vi "PXI-Can Resume From Error.vi"(0 "Ignore local?":bool, 7 "Abort":bool, 11 "error in (no error)":errorcluster) -> (4 "code":i32, 8 "Resume?":bool, 15 "error out":errorcluster)   [LabVIEW 2020]
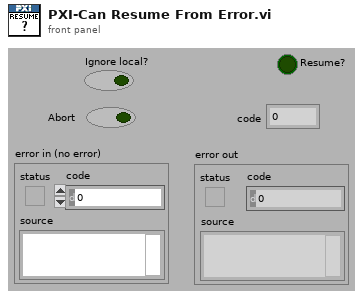
[diagram p1: front panel]
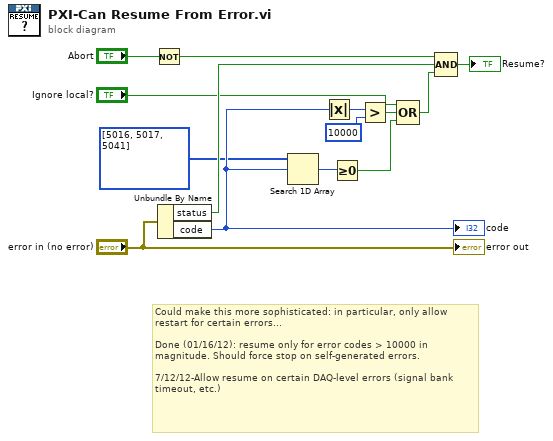
[diagram p0: block diagram]
diagram:
  # "Could make this more sophisticated: in particular, only allow restart for certain errors...\n\nDone (01/16/12): resume only for error codes > 10000 in magnitude. Should force stop on self-generated errors.\n\n7/12/12-Allow resume on certain DAQ-level errors (signal bank timeout, etc.)"
  n1 = Not(x="Abort") -> (.not. x?=w11:bool)
  n2 = Unbundle By Name("error in (no error)") -> ("status"=w12:bool, "code"=w4:i32)
  "code" <- w4
  n3 = Search 1D Array(1D array=i32[] [5016, 5017, 5041], element=w4) -> (index of element=w3:i32)  [unwired: 1 in]
  n4 = Absolute Value(x=w4) -> (abs(x)=w9:i32)
  n5 = Greater Or Equal To 0?(x=w3) -> (x >= 0?=w2:bool)
  n6 = Greater?(x=w9, y=10000) -> (0:w7:bool)
  n7 = Compound Arithmetic op=OR("Ignore local?", w7, w2) -> (w6:bool)
  n8 = Compound Arithmetic op=AND(w11, w12, w6) -> (→"Resume?":bool)
  "error out" <- "error in (no error)"
